vi "Timer.vi"(11 "index":dbl) -> (3 "Time(ms)":sgl)   [LabVIEW 2022 SP3]
panel:
  out "Time":sgl=10.0 format="%#.0f"
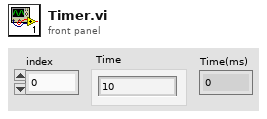
[diagram p1: front panel]
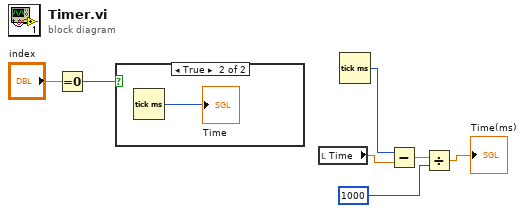
[diagram p0: block diagram]
diagram:
  n1 = Equal To 0?(x="index") -> (x = 0?=w7:bool)
  n2 = case shown="True" w7 {
    frame False {
    }
    frame True {
      n3 = Tick Count (ms)() -> (millisecond timer value=→"Time":u32)
    }
  }
  n4 = local read "Time"() -> (w5:sgl)
  n5 = Tick Count (ms)() -> (millisecond timer value=w6:u32)
  n6 = Subtract(x=w6, y=w5) -> (x-y=w3:sgl)
  n7 = Divide(x=w3, y=1000) -> (x/y=→"Time(ms)":sgl)
